vi "create_batch-custom.vi"(7 "directory":path, 8 "error in (no error)":errorcluster, 11 "configuration":T1) -> (0 "error out":errorcluster, 3 "batch_file":path)   [LabVIEW 2015, in "lv-builder-l3.lvlib"]
uses:
  lv-builder-l3.lvlib
  _controls/l3_configuration.ctl
  <userlib>/antonio-alexander/lv-build/lv-build/lv-build.lvlib
panel:
  out "batch_file":string
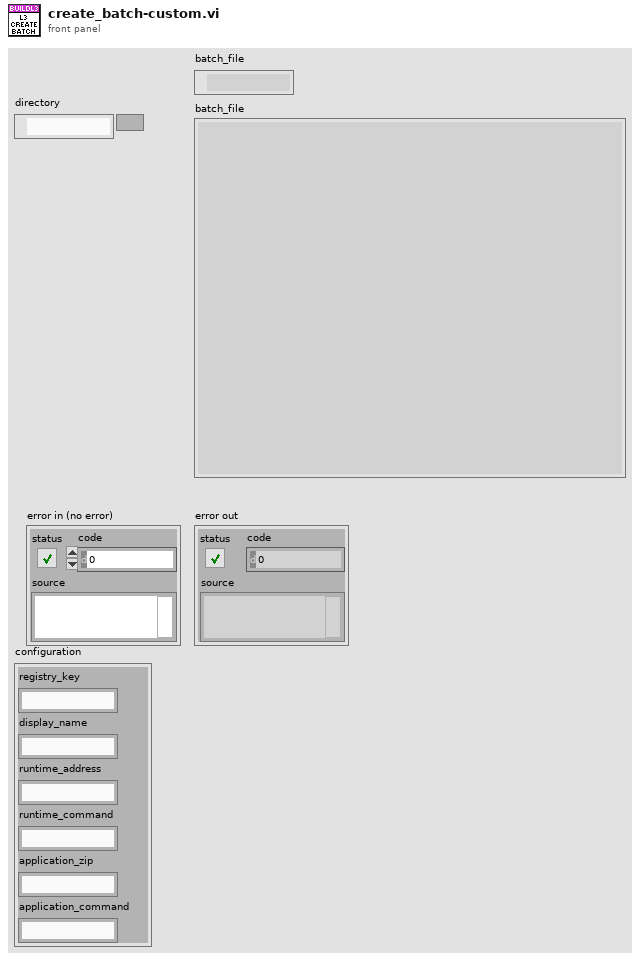
[diagram p1: front panel]
types:
  T1 = typedef "lv-builder-l3.lvlib/l3_configuration.ctl" = cluster{"registry_key":string, "display_name":string, "runtime_address":string, "runtime_command":string, "application_zip":string, "application_command":string}
  T2 = enum16{"open", "replace", "create", "open or create", "replace or create", "replace or create with confirmation"}
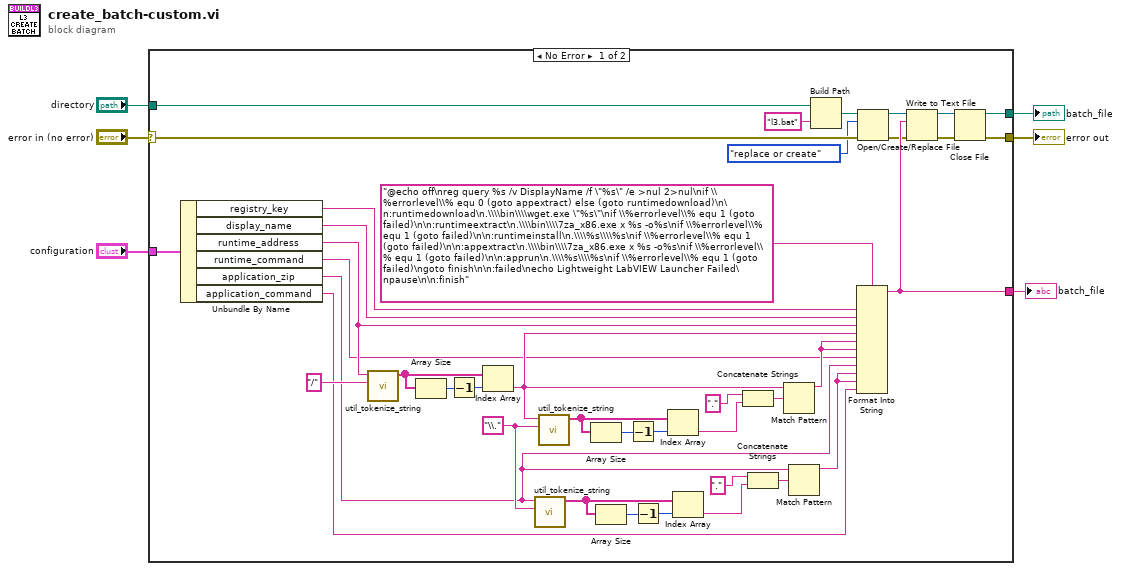
[diagram p0: block diagram]
diagram:
  n1 = case shown="No Error" "error in (no error)" {
    selector: "error in (no error)" -> [w42 w47]
    tunnel: "directory" -> [w46 _]
    tunnel: [w44 w47] -> w2
    tunnel: [w43 _] -> w3
    tunnel: [w23 _] -> w1
    tunnel: "configuration" -> [w7 _]
    frame No Error {
      w25 = "\\." ("delimiter ([\\s\\t\\n\\r]+)")
      n2 = Unbundle By Name(w7) -> ("registry_key"=w13:string, "display_name"=w12:string, "runtime_address"=w11:string, "runtime_command"=w10:string, "application_zip"=w9:string, "application_command"=w8:string)
      n3 = call <userlib>:"util_tokenize_string.vi"("delimiter"="/", "input_string"=w11) -> ("delimited_string []"=w40:string[])  [unwired: 8 in, 1 out]
      n4 = Array Size(array=w40) -> (size(s)=w39:i32)
      n5 = Decrement(x=w39) -> (x-1=w38:i32)
      n6 = Index Array(array=w40, index=w38) -> (element=w21:string)
      n7 = call <userlib>:"util_tokenize_string.vi"("delimiter"=w25, "input_string"=w9) -> ("delimited_string []"=w26:string[])  [unwired: 8 in, 1 out]
      n8 = call <userlib>:"util_tokenize_string.vi"("delimiter"=w25, "input_string"=w21) -> ("delimited_string []"=w32:string[])  [unwired: 8 in, 1 out]
      n9 = Array Size(array=w32) -> (size(s)=w37:i32)
      n10 = Array Size(array=w26) -> (size(s)=w27:i32)
      n11 = Decrement(x=w37) -> (x-1=w36:i32)
      n12 = Decrement(x=w27) -> (x-1=w28:i32)
      n13 = Index Array(array=w32, index=w36) -> (element=w35:string)
      n14 = Index Array(array=w26, index=w28) -> (element=w29:string)
      n15 = Concatenate Strings("." ("string"), w35) -> (w33:string)
      n16 = Concatenate Strings("." ("string"), w29) -> (w31:string)
      n17 = Match Pattern(string=w21, regular expression=w33) -> (before substring=w20:string)  [unwired: 1 in, 3 out]
      n18 = Match Pattern(string=w9, regular expression=w31) -> (before substring=w19:string)  [unwired: 1 in, 3 out]
      n19 = Build Path(base path=w46, name or relative path="l3.bat") -> (appended path=w45:path)
      n20 = Format Into String(format string="@echo off\nreg query %s /v DisplayName /f \"%s\" /e >nul 2>nul\nif \\%errorlevel\\% equ 0 (goto appextract) else (goto runtimedownload)\n\n:runtimedownload\n.\\\\bin\\\\wget.exe \"%s\"\nif \\%errorlevel\\% equ 1 (goto failed)\n\n:runtimeextract\n.\\\\bin\\\\7za_x86.exe x %s -o%s\nif \\%errorlevel\\% equ 1 (goto failed)\n\n:runtimeinstall\n.\\\\%s\\\\%s\nif \\%errorlevel\\% equ 1 (goto failed)\n\n:appextract\n.\\\\bin\\\\7za_x86.exe x %s -o%s\nif \\%errorlevel\\% equ 1 (goto failed)\n\n:apprun\n.\\\\%s\\\\%s\nif \\%errorlevel\\% equ 1 (goto failed)\ngoto finish\n\n:failed\necho Lightweight LabVIEW Launcher Failed\npause\n\n:finish", w13, w12, w11, w21, w20, w20, w10, w9, w19, w19, w8) -> (resulting string=w23:string)  [unwired: 2 in, 1 out]
      n21 = Open/Create/Replace File(file path (use dialog)=w45, error in=w42, operation (0:open)=T2."replace or create") -> (refnum out=w18:refnum<file>, error out=w15:errorcluster)  [unwired: 3 in, 1 out]
      n22 = Write to Text File(file (use dialog)=w18, text=w23, error in=w15) -> (refnum out=w17:refnum<file>, error out=w16:errorcluster)  [unwired: 1 in, 1 out]
      n23 = Close File(refnum=w17, error in=w16) -> (path=w43:path, error out=w44:errorcluster)
    }
    frame Error {
    }
  }
  "error out" <- w2
  "batch_file" <- w3
  "batch_file" <- w1
